vi "Working_I2C Slav_DoSomethinge_WarrenColors.vi"   [LabVIEW 2015]
doc: "This example shows how to send data between 2 Arduino boards using the I2C interface. This is the Slave (receiving) end of the communication. In this example, the Slave registers a callback VI to be run whenever an I2C receive interrupt occurs making this an interrupt driven message handler. When an I2C message comes in, the data is formatted and written to the serial terminal for demo purposes only."
uses:
  <vilib>/Aledyne-TSXperts/Arduino Compatible Compiler for LabVIEW/Code Generator/Arduino APIs/I2C/I2C Mode.ctl
  <vilib>/Aledyne-TSXperts/Arduino Compatible Compiler for LabVIEW/Code Generator/Arduino APIs/Serial/Serial Settings.ctl
  <vilib>/Aledyne-TSXperts/Arduino Compatible Compiler for LabVIEW/Code Generator/Arduino APIs/RGB LED Strip/RGB Strip Mode.ctl
  <vilib>/Aledyne-TSXperts/Arduino Compatible Compiler for LabVIEW/Code Generator/Arduino APIs/Digital/PinDirection.ctl
  Global 3.vi
  <vilib>/Aledyne-TSXperts/Arduino Compatible Compiler for LabVIEW/Arduino Compatible Compiler for LabVIEW.lvlib
panel:
  # "Overview: Demonstrates how to send data between 2 Arduino boards using the I2C interface.  This is the Master (transmitting) end of the communication.  In this example, the Master writes its loop and timing information to the Slave as a String.  When an I2C message comes in, the data is formatted and written to the serial terminal for demo purposes only.\n\nInstructions:\n1. Wire 2 Arduino boards together as shown below.  Connect their SCL lines together and their SDA lines together.  These can appear on different pins depending on which boards are used.  Also note to connect the GND pins of each board together if not powered from the same supply or USB port/hub.\n2.  Open Tools>Arduino Compatible Compiler for LabVIEW in LabVIEW, then select File>Load VI, and select this VI and then Compile and Download.\n3. Once downloaded, open a serial connection to the Slave Arduino board and observe the received data being printed.  Hold the reset button down on the Master and notice that the data stops.  Release the reset and notice the loop number and tick counter restart."
types:
  T1 = typedef "Arduino Compatible Compiler for LabVIEW.lvlib/PinDirection.ctl" = enum16{" INPUT", "OUTPUT", " INPUT_PULLUP"}
  T2 = typedef "Arduino Compatible Compiler for LabVIEW.lvlib/RGB Strip Mode.ctl" = u16
  T3 = typedef "Arduino Compatible Compiler for LabVIEW.lvlib/Serial Settings.ctl" = u16
  T4 = typedef "Arduino Compatible Compiler for LabVIEW.lvlib/I2C Mode.ctl" = enum16{"Master", "Slave"}
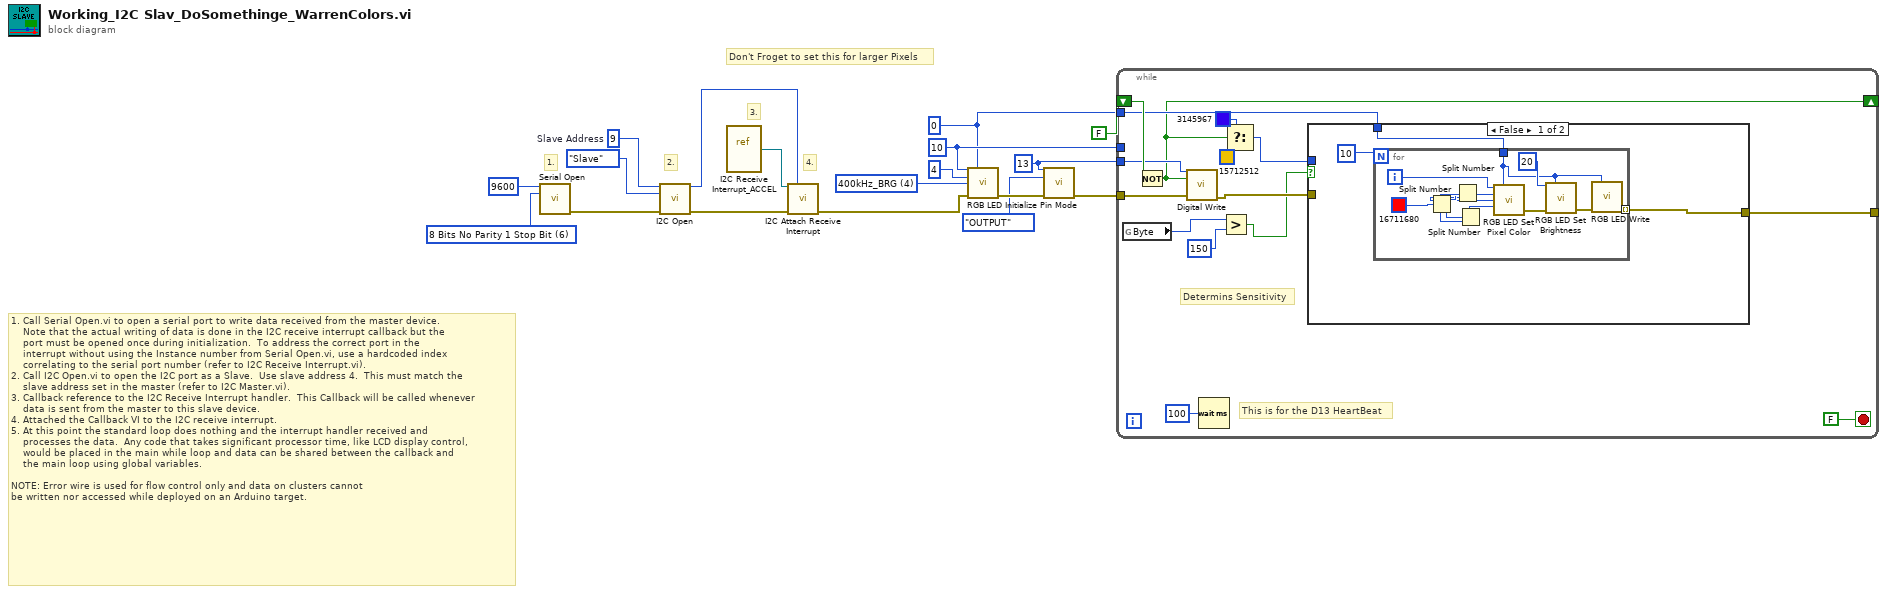
[diagram p0: block diagram]
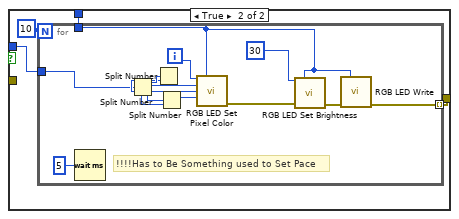
[diagram p2: hidden frame]
diagram:
  w4 = u8 13 ("pin")
  w2 = u8 0 ("Instance")
  w3 = u16 10 ("Number of Pixels")
  w10 = T2 4 items=["400kHz_RGB"=0, "400kHz_GRB"=1, "400kHz_BRG"=4, "800kHz_RGB"=2, "800kHz_GRB"=3, "400kHz_BRG"=6] ("Mode")
  w14 = T3 6 items=["5 Bits No Parity 1 Stop Bit"=0, "6 Bits No Parity 1 Stop Bit"=2, "7 Bits No Parity 1 Stop Bit"=4, "8 Bits No Parity 1 Stop Bit"=6, "5 Bits No Parity 2 Stop Bits"=8, "6 Bits No Parity 2 Stop Bits"=10, "7 Bits No Parity 2 Stop Bits"=12, "8 Bits No Parity 2 Stop Bits"=14, "5 Bits Even Parity 1 Stop Bits"=32, "6 Bits Even Parity 1 Stop Bits"=34, "7 Bits Even Parity 1 Stop Bits"=36, "8 Bits Even Parity 1 Stop Bits"=38, "5 Bits Even Parity 2 Stop Bits"=40, "6 Bits Even Parity 2 Stop Bits"=42, "7 Bits Even Parity 2 Stop Bits"=44, "8 Bits Even Parity 2 Stop Bits"=46, "5 Bits Odd Parity 1 Stop Bits"=48, "6 Bits Odd Parity 1 Stop Bits"=50, "7 Bits Odd Parity 1 Stop Bits"=52, "8 Bits Odd Parity 1 Stop Bits"=54, "5 Bits Odd Parity 2 Stop Bits"=56, "6 Bits Odd Parity 2 Stop Bits"=58, "7 Bits Odd Parity 2 Stop Bits"=60, "8 Bits Odd Parity 2 Stop Bits"=62] ("Serial Settings")
  w17 = u8 9  # Slave Address
  # "Don't Froget to set this for larger Pixels"
  # "4."
  # "3."
  # "2."
  # "1."
  # "1. Call Serial Open.vi to open a serial port to write data received from the master device.\n    Note that the actual writing of data is done in the I2C receive interrupt callback but the\n    port must be opened once during initialization.  To address the correct port in the\n    interrupt without using the Instance number from Serial Open.vi, use a hardcoded index\n    correlating to the serial port number (refer to I2C Receive Interrupt.vi).\n2. Call I2C Open.vi to open the I2C port as a Slave.  Use slave address 4.  This must match the\n    slave address set in the master (refer to I2C Master.vi).\n3. Callback reference to the I2C Receive Interrupt handler.  This Callback will be called whenever\n    data is sent from the master to this slave device.\n4. Attached the Callback VI to the I2C receive interrupt.\n5. At this point the standard loop does nothing and the interrupt handler received and\n    processes the data.  Any code that takes significant processor time, like LCD display control,\n    would be placed in the main while loop and data can be shared between the callback and\n    the main loop using global variables.\n\nNOTE: Error wire is used for flow control only and data on clusters cannot\nbe written nor accessed while deployed on an Arduino target."
  n1 = call <vilib>:"Serial Open.vi"("Speed"=u32 9600, "Serial Settings"=w14) -> ("error out"=w13:errorcluster)  [unwired: 12 in, 1 out]
  n2 = call <vilib>:"I2C Open.vi"("Slave Address"=w17, "Mode"=I2C_Mode."Slave", "error in (no error)"=w13) -> ("Interface"=w12:u8, "error out"=w16:errorcluster)  [unwired: 11 in]
  n3 = vi-ref "I2C Receive Interrupt_ACCEL.vi"() -> (w11:refnum<vi>)
  n4 = call <vilib>:"I2C Attach Receive Interrupt.vi"("VI Reference"=w11, "Interface"=w12, "error in (no error)"=w16) -> ("error out"=w1:errorcluster)  [unwired: 12 in]
  n5 = call <vilib>:"RGB LED Initialize.vi"("Number of Pixels"=w3, "Instance"=w2, "Pin"=u8 4, "Mode"=w10, "error in (no error)"=w1) -> ("error out"=w8:errorcluster)  [unwired: 10 in]
  n6 = call <vilib>:"Pin Mode.vi"("pin"=w4, "direction"=PinDirection."OUTPUT", "error in (no error)"=w8) -> ("error out"=w6:errorcluster)  [unwired: 12 in]
  n7 = while {
    tunnel: w6 -> [w33]
    shift-right: [w20] -> _
    shift-left: FALSE -> [w32]
    tunnel: w4 -> [w31]
    tunnel: w3 -> [_]
    tunnel: w2 -> [w28]
    tunnel: [w26] -> _
    stop <- FALSE stop-if-true
    # "Determins Sensitivity"
    # "This is for the D13 HeartBeat"
    n8 = global read "Global 3.vi" "Byte"() -> (w25:u8)
    n9 = Not(x=w32) -> (.not. x?=w20:bool)
    n10 = call <vilib>:"Digital Write.vi"("pin"=w31, "state"=w20, "error in (no error)"=w33) -> ("error out"=w27:errorcluster)  [unwired: 12 in]
    n11 = Wait (ms)(milliseconds to wait=u32 100) -> ()  [unwired: 1 out]
    n12 = Greater?(x=w25, y=u8 150) -> (0:w23:bool)
    n13 = Select(t=u32 3145967, s=w20, f=u32 15712512) -> (s? t:f=w19:u32)
    n14 = case shown="False" w23 {
      tunnel: w28 -> [w36 w52]
      tunnel: w27 -> [_ _]
      tunnel: [w34 w50] -> w26
      tunnel: w19 -> [_ w49]
      frame False {
        n15 = for {
          N: 10 -> [_]
          tunnel: w36 -> [w38]
          tunnel: [w39] -> w34 mode=indexing
          i -> [w37]
          n16 = Split Number(x=u32 16711680) -> (hi(x)=w42:u16, lo(x)=w43:u16)
          n17 = Split Number(x=w42) -> (lo(x)=w41:u8)  [unwired: 1 out]
          n18 = Split Number(x=w43) -> (hi(x)=w40:u8, lo(x)=w44:u8)
          n19 = call <vilib>:"RGB LED Set Pixel Color.vi"("Pixel"=w37, "Instance"=w38, "Red"=w44, "Green"=w41, "Blue"=w40) -> ("error out"=w48:errorcluster)  [unwired: 10 in]
          n20 = call <vilib>:"RGB LED Set Brightness.vi"("Brightness"=u8 20, "Instance"=w38, "error in (no error)"=w48) -> ("error out"=w46:errorcluster)  [unwired: 12 in]
          n21 = call <vilib>:"RGB LED Write.vi"("Instance"=w38, "error in (no error)"=w46) -> ("error out"=w39:errorcluster)  [unwired: 13 in]
        }
      }
      frame True {
        n22 = for {
          N: 10 -> [_]
          tunnel: w52 -> [w58]
          tunnel: [w57] -> w50 mode=indexing
          tunnel: w49 -> [w53]
          i -> [w56]
          # "!!!!Has to Be Something used to Set Pace"
          n23 = Wait (ms)(milliseconds to wait=u32 5) -> ()  [unwired: 1 out]
          n24 = Split Number(x=w53) -> (hi(x)=w62:u16, lo(x)=w63:u16)
          n25 = Split Number(x=w62) -> (lo(x)=w61:u8)  [unwired: 1 out]
          n26 = Split Number(x=w63) -> (hi(x)=w60:u8, lo(x)=w64:u8)
          n27 = call <vilib>:"RGB LED Set Pixel Color.vi"("Pixel"=w56, "Instance"=w58, "Red"=w64, "Green"=w61, "Blue"=w60) -> ("error out"=w54:errorcluster)  [unwired: 10 in]
          n28 = call <vilib>:"RGB LED Set Brightness.vi"("Brightness"=u8 30, "Instance"=w58, "error in (no error)"=w54) -> ("error out"=w65:errorcluster)  [unwired: 12 in]
          n29 = call <vilib>:"RGB LED Write.vi"("Instance"=w58, "error in (no error)"=w65) -> ("error out"=w57:errorcluster)  [unwired: 13 in]
        }
      }
    }
  }
